vi "Replace_String.vi"(11 "input string":string) -> (3 "result string":string)   [LabVIEW 2021]
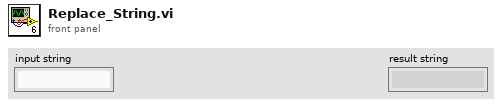
[diagram p1: front panel]
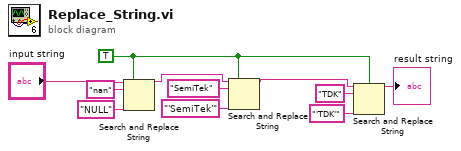
[diagram p0: block diagram]
diagram:
  w3 = TRUE ("replace all? (F)")
  n1 = Search and Replace String(replace all?=w3, input string="input string", search string="nan", replace string="NULL" ("replace string (\"\")")) -> (result string=w7:string)  [unwired: 4 in, 3 out]
  n2 = Search and Replace String(replace all?=w3, input string=w7, search string="SemiTek", replace string="'SemiTek'" ("replace string (\"\")")) -> (result string=w4:string)  [unwired: 4 in, 3 out]
  n3 = Search and Replace String(case sensitive?=w3, input string=w4, search string="TDK", replace string="'TDK'" ("replace string (\"\")")) -> (result string=→"result string":string)  [unwired: 4 in, 3 out]
